vi "Configure Channel (Pulse Normal).vi"(0 "VISA resource name":refnum<visa-resource-name>, 1 "Channel (0001)":string="0001", 2 "Enable Channel (True)":bool=TRUE, 3 "Range (0 : Level)":i32(ring) items=["Level", "Contact"], 4 "Chattering filter (On)":bool=TRUE, 5 "Span":T1={"Lower Span (0)"=0, "Upper Span (200000)"=200000} {"Upper Span (200000)" min=0 max=200000 step=1; "Lower Span (0)" min=0 max=200000 step=1}, 7 "error in (no error)":errorcluster) -> (20 "VISA resource name out":refnum<visa-resource-name>, 21 "Channel":string, 27 "error out":errorcluster)   [LabVIEW 2020, in "Yokogawa GX Series.lvlib"]
doc: "Sets the input range of Pulse input channels.\n\nCommand: SRangePulse"
uses:
  <instrlib>/Yokogawa GX Series/Yokogawa GX Series.lvlib
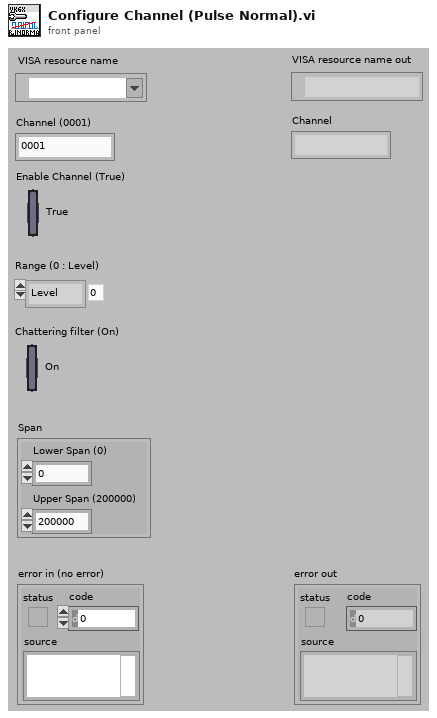
[diagram p1: front panel]
types:
  T1 = cluster{"Lower Span (0)":i32, "Upper Span (200000)":i32}
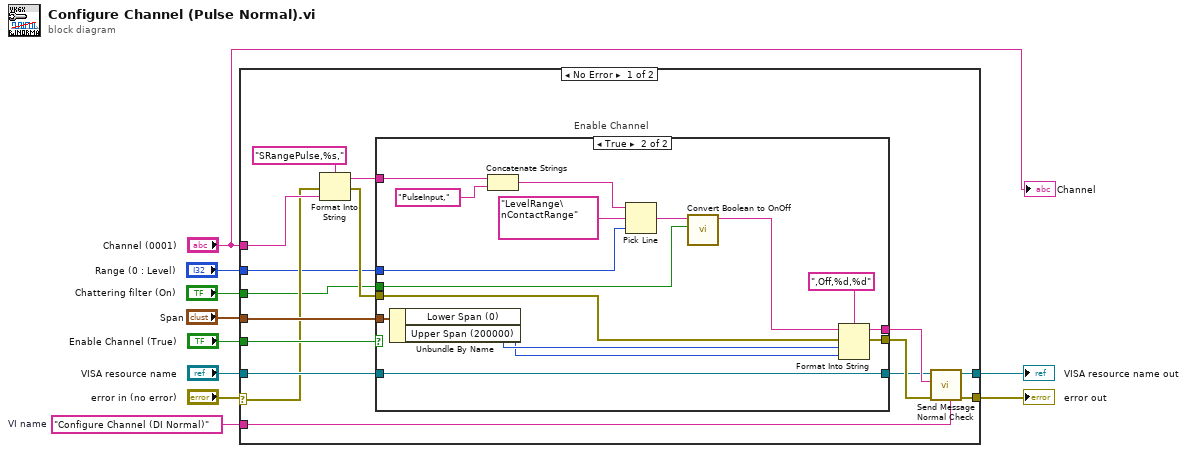
[diagram p0: block diagram]
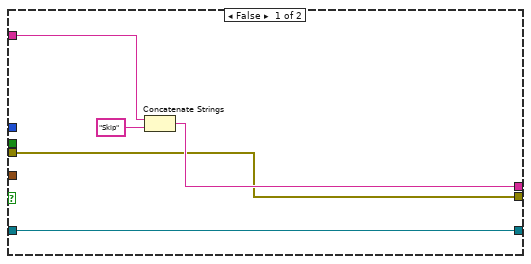
[diagram p2: hidden frame]
diagram:
  w7 = "Configure Channel (DI Normal)"  # VI name
  n1 = case shown="No Error" "error in (no error)" {
    selector: "error in (no error)" -> [w13 w48]
    tunnel: "Enable Channel (True)" -> [w23 _]
    tunnel: [w22 w49] -> w9
    tunnel: [w21 w48] -> w8
    tunnel: w7 -> [w18 _]
    tunnel: "Span" -> [w17 _]
    tunnel: "VISA resource name" -> [w16 w49]
    tunnel: "Channel (0001)" -> [w14 _]
    tunnel: "Range (0 : Level)" -> [w12 _]
    tunnel: "Chattering filter (On)" -> [w11 _]
    frame No Error {
      # "Enable Channel"
      n2 = Format Into String(format string="SRangePulse,%s,", error in=w13, w14) -> (resulting string=w24:string, error out=w25:errorcluster)  [unwired: 1 in]
      n3 = case shown="True" w23 {
        tunnel: w25 -> [w28 w46]
        tunnel: [w28 w45] -> w20
        tunnel: w24 -> [w29 w39]
        tunnel: [w30 w44] -> w19
        tunnel: w17 -> [_ w43]
        tunnel: w16 -> [w27 w42]
        tunnel: [w27 w42] -> w15
        tunnel: w12 -> [_ w35]
        tunnel: w11 -> [_ w32]
        frame False {
          n4 = Concatenate Strings(w29, "Skip") -> (w30:string)
        }
        frame True {
          n5 = Unbundle By Name(w43) -> ("Lower Span (0)"=w41:i32, "Upper Span (200000)"=w40:i32)
          n6 = Concatenate Strings(w39, "PulseInput,") -> (w37:string)
          n7 = Pick Line(string ("")=w37, multi-line string="LevelRange\nContactRange", line index=w35) -> (output string=w34:string)
          n8 = call <instrlib>:"Convert Boolean to OnOff.vi"("On/Off"=w32, "Initial String (\"\")"=w34) -> ("Resulting String"=w33:string)  [unwired: 9 in]
          n9 = Format Into String(format string=",Off,%d,%d", initial string=w33, error in=w46, w41, w40) -> (resulting string=w44:string, error out=w45:errorcluster)
        }
      }
      n10 = call <instrlib>:"Send Message Normal Check.vi"("Source (\"\")"=w18, "error in (no error)"=w20, "Send Message (\"\")"=w19, "VISA resource name"=w15) -> ("error out"=w21:errorcluster, "VISA resource name out"=w22:refnum<visa-resource-name>)  [unwired: 2 in, 4 out]
    }
    frame Error {
    }
  }
  "error out" <- w8
  "VISA resource name out" <- w9
  "Channel" <- "Channel (0001)"
